vi "Find Next Visible Trees.vi"(0 "Next Trees":i32[](array[numeric]), 1 "Current Tree":i32) -> (2 "#Next Visible Trees":i32)   [LabVIEW 2020, in "AoC 2022.lvlib"]
uses:
  AoC 2022.lvlib
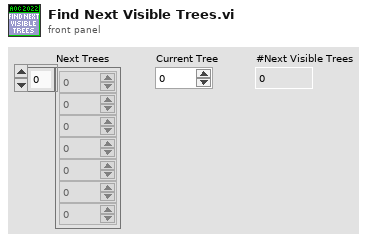
[diagram p1: front panel]
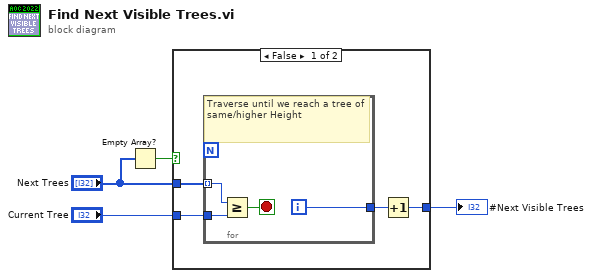
[diagram p0: block diagram]
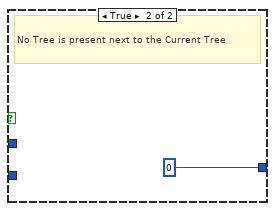
[diagram p2: hidden frame]
diagram:
  n1 = Empty Array?(array="Next Trees") -> (empty?=w1:bool)
  n2 = case shown="False" w1 {
    tunnel: "Current Tree" -> [w8 _]
    tunnel: "Next Trees" -> [w7 _]
    tunnel: [w5 0] -> w3
    frame False {
      n3 = for {
        tunnel: w8 -> [w12]
        tunnel: w7 -> [w11] mode=indexing
        tunnel: [w9] -> w6
        i -> [w9]
        stop <- w10 stop-if-true
        # "Traverse until we reach a tree of same/higher Height"
        n4 = Greater Or Equal?(x=w11, y=w12) -> (x >= y?=w10:bool)
      }
      n5 = Increment(x=w6) -> (x+1=w5:i32)
    }
    frame True {
      # "No Tree is present next to the Current Tree"
    }
  }
  "#Next Visible Trees" <- w3
